vi "Actor Core.vi"(8 "error in":errorcluster, 11 "Root Actor in":refnum<class "Root Actor.lvclass">) -> (0 "error out":errorcluster, 3 "Actor out":refnum<class "Actor.lvclass">)   [LabVIEW 2020, in "Nested Actor.lvlib" / "Root Actor.lvclass"]
doc: "(<B>Filename</B>: Actor Framework.lvlib:Actor.lvclass:Actor Core.vi)\n\nReceives messages to the actor, reacts to them, and initiates any error handling that may shut the actor down.\n\nDescendant classes may override this VI to append parallel tasks for the actor to complete while it handles messages. Overrides use the Call Parent Class Method node."
uses:
  Root Actor.lvclass
  C:/Program Files (x86)/National Instruments/LabVIEW 2020/vi.lib/ActorFramework/Actor/Actor.lvclass
  <vilib>/ActorFramework/Actor/Actor.lvclass
  <vilib>/ActorFramework/Actor/Actor.lvclass/Actor.ctl
  <vilib>/ActorFramework/Message Enqueuer/Message Enqueuer.lvclass/Message Enqueuer.ctl
  Root Actor.lvclass/Root Actor.ctl
  Root Actor Messages/Tx Content Msg/Tx Nested Content Msg.lvclass/Tx Nested Content Msg.ctl
  <vilib>/ActorFramework/Message Enqueuer/Init from Existing Queue.vi
  <vilib>/ActorFramework/Message Enqueuer/Enqueue.vi
  <vilib>/ActorFramework/Stop Msg/Stop Msg.lvclass
  C:/Program Files (x86)/National Instruments/LabVIEW 2020/vi.lib/ActorFramework/Message/Message.lvclass
  Root Actor Messages/Launch Nested Msg/Launch Nested Msg.lvclass
  Root Actor Messages/Tx Content Msg/Tx Nested Content Msg.lvclass
  <vilib>/ActorFramework/Message Priority Queue/Priority Enqueue.vi
  <vilib>/ActorFramework/Message Enqueuer/Message Enqueuer.lvclass
panel:
  out "Rcv From Nested":string
  in  "BT_Stop":bool
  in  "BT_Launch":bool
  in  "Content":string
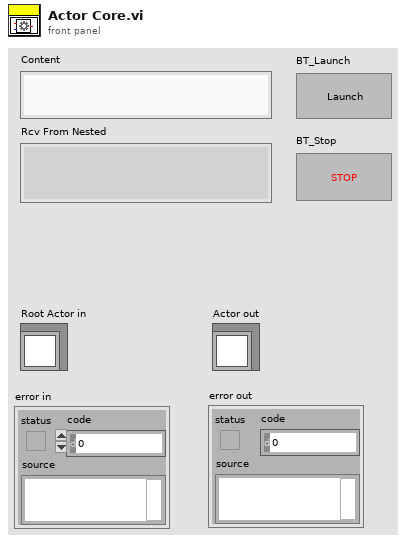
[diagram p1: front panel]
types:
  T1 = cluster{"Stop Event":refnum<user-event>, "Rcv Event":refnum<user-event>}
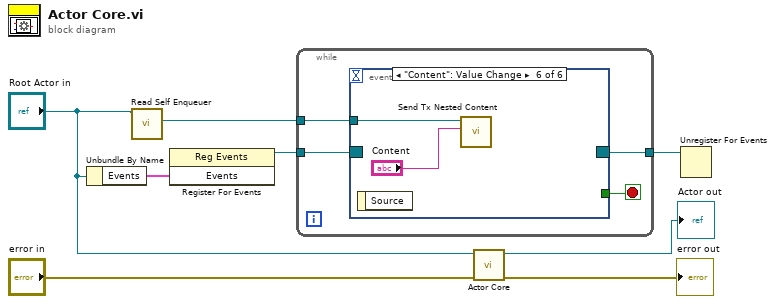
[diagram p0: block diagram]
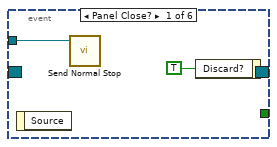
[diagram p2: hidden frame]
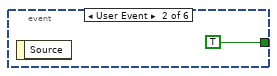
[diagram p3: hidden frame]
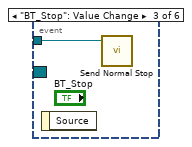
[diagram p4: hidden frame]
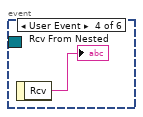
[diagram p5: hidden frame]
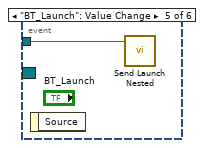
[diagram p6: hidden frame]
diagram:
  n1 = Unbundle By Name("Root Actor in") -> ("Events"=w5:T1)
  n2 = call <vilib>:"Read Self Enqueuer.vi"("Actor"="Root Actor in") -> ("Self Enqueuer"=w1:refnum<class "Message Enqueuer.lvclass">)  [unwired: 10 in]
  n3 = register-events(w5) -> (reference out=w4:refnum<event-registration>)  [unwired: 2 in, 1 out]
  n4 = while {
    tunnel: w4 -> [w12]
    tunnel: [w11] -> w3
    tunnel: w1 -> [w10]
    stop <- w9 stop-if-true
    n5 = event shown="[5] \"Content\": Value Change" {
      selector: w12 -> [_ _ _ _ _ _]
      dyn-events: [_ _ _ _ _ _] -> w11
      timeout: _ -> [_ _ _ _ _ _]
      tunnel: w10 -> [w13 _ w16 _ w18 w20]
      tunnel: [_ TRUE _ _ _ _] -> w9
      event Panel Close? {
        n6 = event-data() -> ()  [unwired: 1 in, 1 out]
        n7 = call <vilib>:"Send Normal Stop.vi"("Message Enqueuer"=w13) -> ()  [unwired: 10 in, 1 out]
        n8 = event-data("Discard?"=TRUE) -> ()  [unwired: 1 in, 1 out]
      }
      event User Event {
        n9 = event-data() -> ()  [unwired: 1 in, 1 out]
      }
      event "BT_Stop": Value Change {
        n10 = event-data() -> ()  [unwired: 1 in, 1 out]
        n11 = call <vilib>:"Send Normal Stop.vi"("Message Enqueuer"=w16) -> ()  [unwired: 10 in, 1 out]
      }
      event User Event {
        n12 = event-data() -> ("Rcv"=→"Rcv From Nested":string)  [unwired: 1 in]
      }
      event "BT_Launch": Value Change {
        n13 = event-data() -> ()  [unwired: 1 in, 1 out]
        n14 = call "Send Launch Nested.vi"("Message Enqueuer"=w18) -> ()  [unwired: 9 in, 2 out]
      }
      event "Content": Value Change {
        n15 = event-data() -> ()  [unwired: 1 in, 1 out]
        n16 = call "Send Tx Nested Content.vi"("Content"="Content", "Message Enqueuer"=w20) -> ()  [unwired: 8 in, 2 out]
      }
    }
  }
  n17 = call-parent "Actor Core.vi"("error in"="error in", "Actor in"="Root Actor in") -> ("error out"=→"error out":errorcluster, "Actor out"=→"Actor out":refnum<class "Actor.lvclass">)  [unwired: 8 in]
  n18 = Unregister For Events(event registration refnum=w3) -> ()  [unwired: 1 in, 1 out]
